vi "SV Close XLS.vi"(2 "error in (no error)":errorcluster, 3 "Save? (F)":bool, 4 "Refnum Cluster In":T1, 5 "path 2":path) -> (0 "error out":errorcluster, 1 "Refnum Cluster Out":T2)   [LabVIEW 2010]
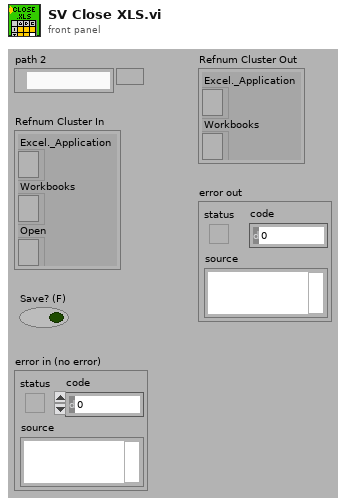
[diagram p1: front panel]
types:
  T1 = cluster{"Excel._Application":refnum<k7>, "Workbooks":refnum<k7>, "Open":refnum<k7>}
  T2 = cluster{"Excel._Application":refnum<k7>, "Workbooks":refnum<k7>}
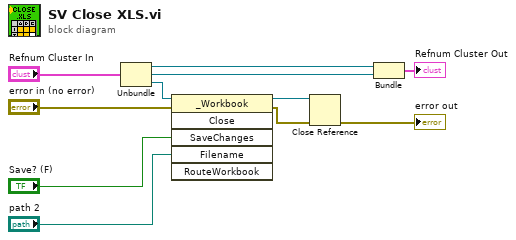
[diagram p0: block diagram]
diagram:
  n1 = Unbundle("Refnum Cluster In") -> ("Excel._Application"=w6:refnum<k7>, "Workbooks"=w7:refnum<k7>, "Open"=w8:refnum<k7>)
  n2 = invoke class="_Workbook" method="Close"(reference=w8, error in="error in (no error)", "SaveChanges"="Save? (F)", "Filename"="path 2") -> (reference out=w2:refnum<k7>, error out=w1:errorcluster)  [unwired: 2 in, 4 out]
  n3 = Close Reference(reference=w2, error in (no error)=w1) -> (error out=→"error out":errorcluster)
  n4 = Bundle("Excel._Application"=w6, "Workbooks"=w7) -> (→"Refnum Cluster Out":T2)  [unwired: 1 in]
